vi "ReadWriteAttributeOld.vi"(0 "reference in":refnum<class "G#MethodTemplates.lvclass">, 5 "error in (no error)":errorcluster) -> (14 "reference out":refnum<class "G#MethodTemplates.lvclass">, 19 "error out":errorcluster)   [LabVIEW 2020, in "G#MethodTemplates.lvclass"]
uses:
  G#MethodTemplates.lvclass
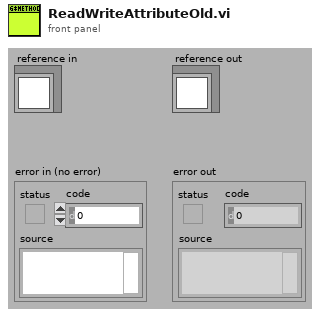
[diagram p1: front panel]
types:
  T1 = typedef "G#MethodTemplates.lvclass/ObjectAttributes.ctl" = cluster{"Numeric":dbl}
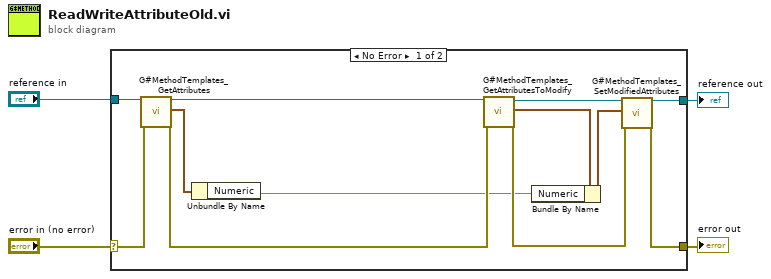
[diagram p0: block diagram]
diagram:
  n1 = case shown="No Error" "error in (no error)" {
    selector: "error in (no error)" -> [w10 w18]
    tunnel: [w14 w18] -> w3
    tunnel: [w13 w17] -> w1
    tunnel: "reference in" -> [w11 w17]
    frame No Error {
      n2 = call "G#MethodTemplates_GetAttributes.vi"("reference in"=w11, "error in (no error)"=w10) -> ("reference out"=w8:refnum<class "G#MethodTemplates.lvclass">, "attributes"=w7:T1, "error out"=w9:errorcluster)  [unwired: 14 in, 1 out]
      n3 = Unbundle By Name(w7) -> ("Numeric"=w6:dbl)
      n4 = call "G#MethodTemplates_GetAttributesToModify.vi"("reference in"=w8, "error in (no error)"=w9) -> ("reference out"=w15:refnum<class "G#MethodTemplates.lvclass">, "attributes"=w16:T1, "error out"=w12:errorcluster)  [unwired: 13 in, 2 out]
      n5 = Bundle By Name(cluster=w16, "Numeric"=w6) -> (w5:T1)
      n6 = call "G#MethodTemplates_SetModifiedAttributes.vi"("reference in"=w15, "attributes"=w5, "error in (no error)"=w12) -> ("reference out"=w13:refnum<class "G#MethodTemplates.lvclass">, "error out"=w14:errorcluster)  [unwired: 15 in]
    }
    frame Error {
    }
  }
  "error out" <- w3
  "reference out" <- w1
